vi "test - EventHandler-Change Order By Enter Key.vi"() -> ()   [LabVIEW 2017]
panel:
  in  "cancel":bool
  in  "ok":bool
  in  "Enum":enum16{"a", "b", "cd", "d"}(ring)
  in  "password":string
  in  "String 2":string
  in  "String":string
  # "#NOTE\nyou can switch orders by enter key"
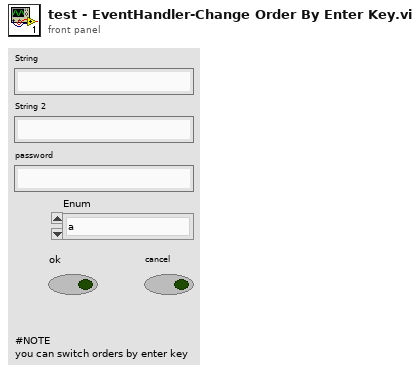
[diagram p1: front panel]
types:
  T1 = typedef "eventvkey.ctl" = enum16{"ASCII", "Enter", "Return", "Shift", "Ctrl", "Alt", "Cmd", "Opt", "Caps", "NumLock", "Clear", "Break", "Up", "Down", "Left", "Right", "Insert", "Delete", "Home", "End", "PageUp", "PageDown", "Escape", "Help", "Pause", "ScrollLock", "F1", "F2", "F3", "F4", "F5", "F6", "F7", "F8", "F9", "F10", "F11", "F12", "F13", "F14", "F15", "F16", "F17", "F18", "F19", "F20", "F21", "F22", "F23", "F24", "Play", "VolumeUp", "VolumeDown", "Mute", "Two Byte Char"}
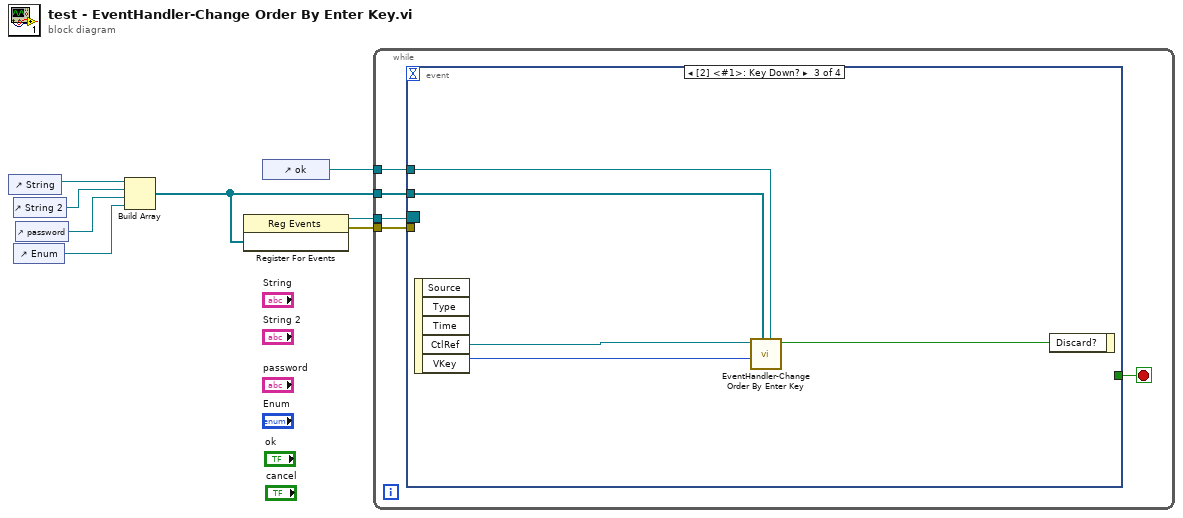
[diagram p0: block diagram]
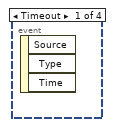
[diagram p2: hidden frame]
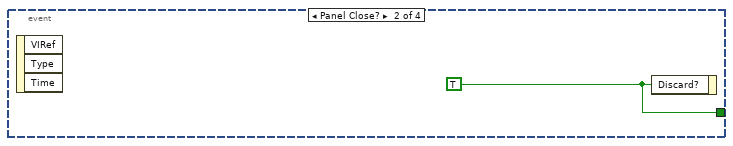
[diagram p3: hidden frame]
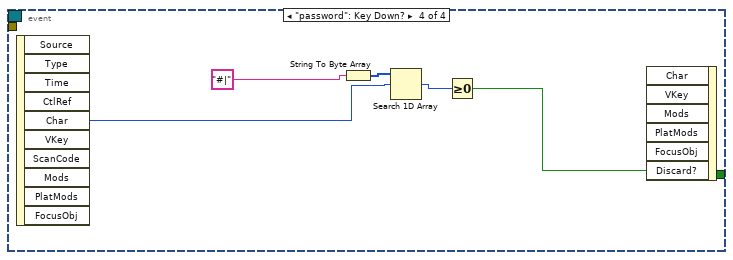
[diagram p4: hidden frame]
diagram:
  n1 = control-ref of="String"() -> (w5:refnum<vi>)
  n2 = control-ref of="String 2"() -> (w4:refnum<vi>)
  n3 = control-ref of="Enum"() -> (w2:refnum<vi>)
  n4 = control-ref of="password"() -> (w3:refnum<vi>)
  n5 = Build Array(w5, w4, w3, w2) -> (w1:refnum<vi>[])
  n6 = register-events(w1) -> (reference out=w7:refnum<event-registration>, error out=w8:errorcluster)  [unwired: 2 in]
  n7 = control-ref of="ok"() -> (w6:refnum<vi>)
  n8 = while {
    tunnel: w8 -> [w12]
    tunnel: w7 -> [w11]
    tunnel: w1 -> [w10]
    tunnel: w6 -> [w9]
    stop <- w13 stop-if-true
    n9 = event shown="[2] <#1>: Key Down?" {
      selector: w11 -> [_ _ _ _]
      dyn-events: _ -> [_ _ _ _]
      timeout: _ -> [_ _ _ _]
      tunnel: [_ w14 _ _] -> w13
      tunnel: w12 -> [_ _ _ _]
      tunnel: w10 -> [_ _ w18 _]
      tunnel: w9 -> [_ _ w17 _]
      event Timeout {
        n10 = event-data() -> ()  [unwired: 1 in, 3 out]
      }
      event Panel Close? {
        w14 = TRUE ("Discard?")
        n11 = event-data() -> ()  [unwired: 1 in, 3 out]
        n12 = event-data("Discard?"=w14) -> ()  [unwired: 1 in, 1 out]
      }
      event Key Down? {
        n13 = event-data() -> ("CtlRef"=w16:refnum<vi>, "VKey"=w15:T1)  [unwired: 1 in, 3 out]
        n14 = call "EventHandler-Change Order By Enter Key.vi"("Next Ctrl"=w17, "Controls for changing order"=w18, "VKey"=w15, "Event Control"=w16) -> ("Discard?"=w19:bool)  [unwired: 7 in]
        n15 = event-data("Discard?"=w19) -> ()  [unwired: 1 in, 1 out]
      }
      event "password": Key Down? {
        n16 = event-data() -> ("Char"=w22:i16)  [unwired: 1 in, 9 out]
        n17 = String To Byte Array(string="#|") -> (unsigned byte array=w23:u8[])
        n18 = Search 1D Array(1D array=w23, element=w22) -> (index of element=w21:i32)  [unwired: 1 in]
        n19 = Greater Or Equal To 0?(x=w21) -> (x >= 0?=w20:bool)
        n20 = event-data("Discard?"=w20) -> ()  [unwired: 6 in, 1 out]
      }
    }
  }
